vi "GetType.vi"(8 "error in (no error)":errorcluster, 11 "Configure DisLevel Msg":refnum<class "Configure DisLevel Msg.lvclass">) -> (0 "error out":errorcluster, 2 "Data Sample":variant, 3 "Configure DisLevel Msg":refnum<class "Configure DisLevel Msg.lvclass">)   [LabVIEW 2015, in "CS++MCS.lvlib" / "Configure DisLevel Msg.lvclass"]
uses:
  Configure DisLevel Msg.lvclass
  Configure DisLevel Msg.lvclass/Configure DisLevel Msg.ctl
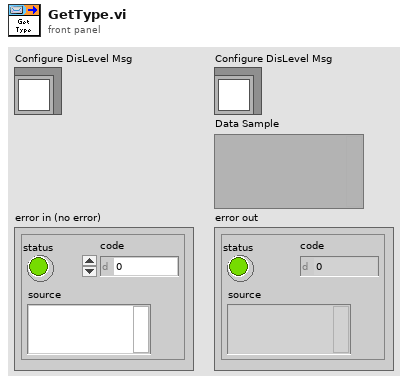
[diagram p1: front panel]
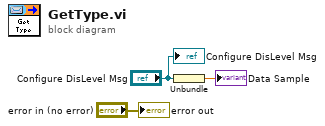
[diagram p0: block diagram]
diagram:
  n1 = Unbundle("Configure DisLevel Msg") -> (→"Data Sample":dbl[unit])
  "error out" <- "error in (no error)"
  "Configure DisLevel Msg" <- "Configure DisLevel Msg"
